vi "GrapgicalLec2.vi"() -> ()   [LabVIEW 2018]
panel:
  in  "Stop Button":bool
  out "String 3":string
  in  "a":dbl
  in  "stop 2":bool
  out "Boolean 5":bool
  out "Boolean 4":bool
  in  "LED 2":bool
  in  "LED 1":bool
  in  "stop":bool
  out "Boolean 2":bool
  in  "Boolean":bool
  out "XY Graph 2":cluster{dbl[], dbl[]}(graph)
  out "XY Graph":cluster{dbl[], dbl[]}(graph)
  out "1 root":bool
  out "2 roots":bool
  out "String":string
  in  "Numeric":dbl
  out "?":dbl
  in  "Focal Length":dbl
  in  "Polarization":dbl(knob) min=0.0 max=90.0 step=5.0 scale=0.0..90.0
  in  "Wavelength":dbl
  in  "Numeric Aperature":dbl
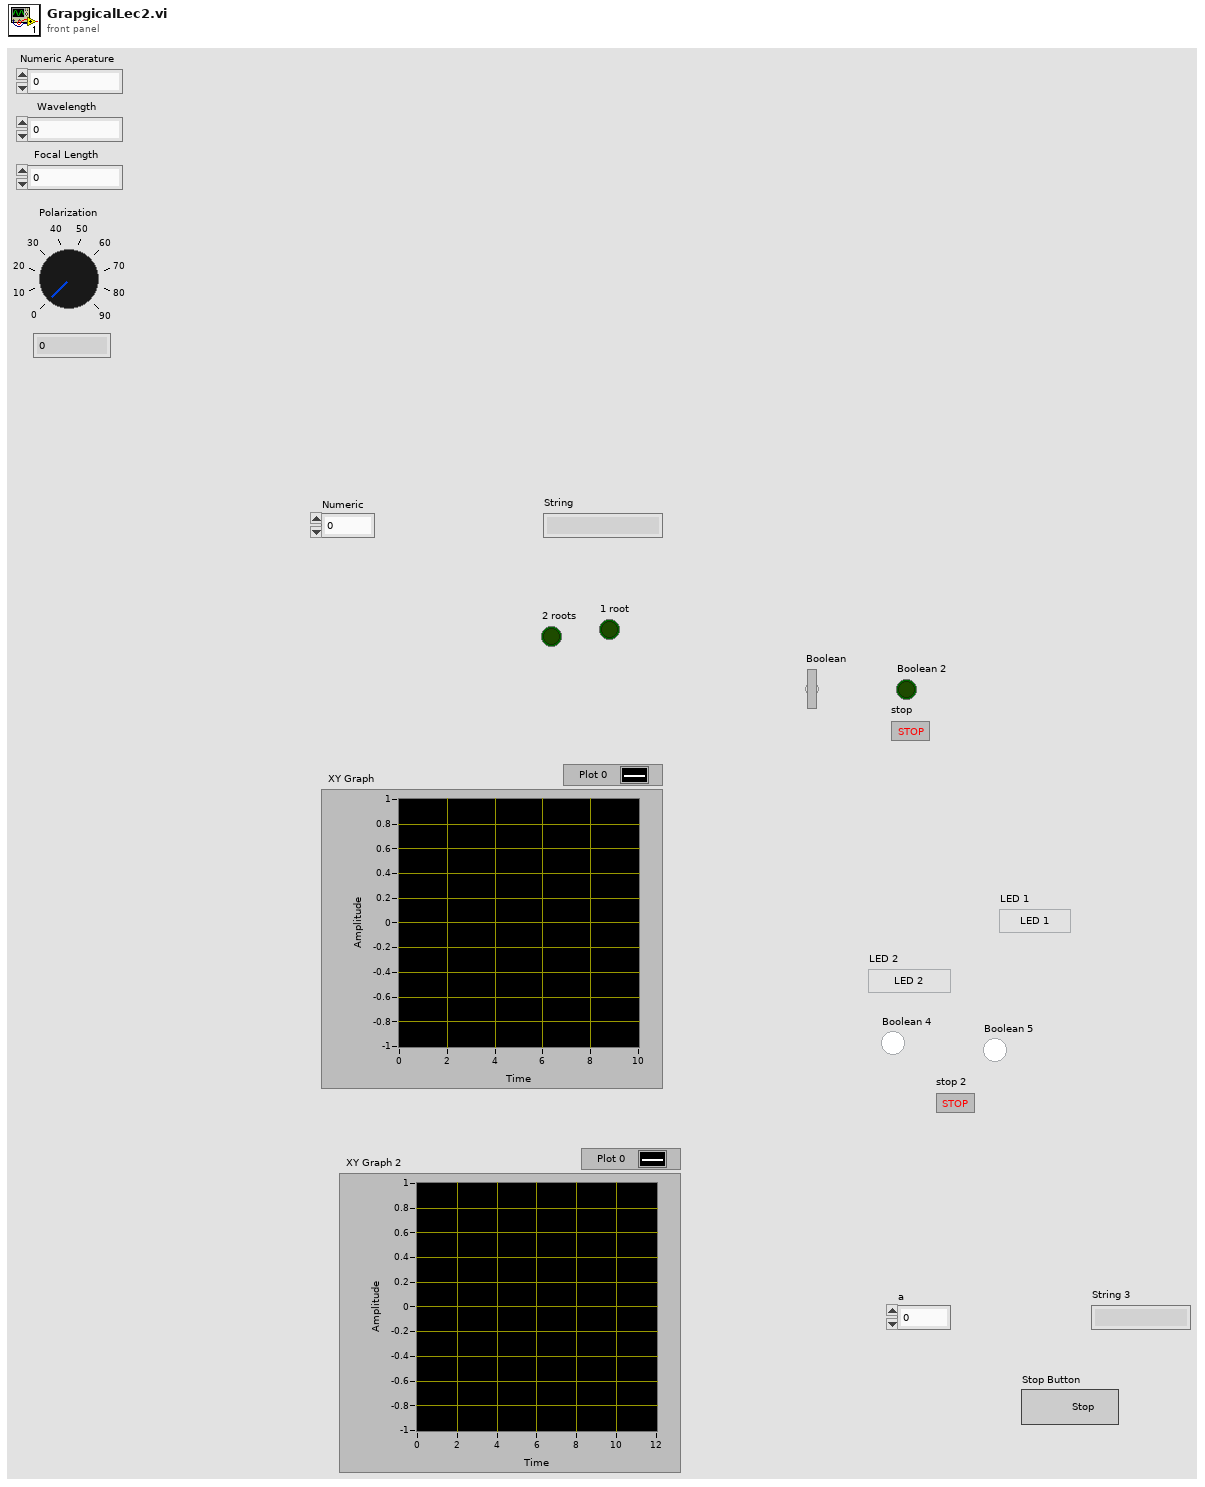
[diagram p1: front panel]
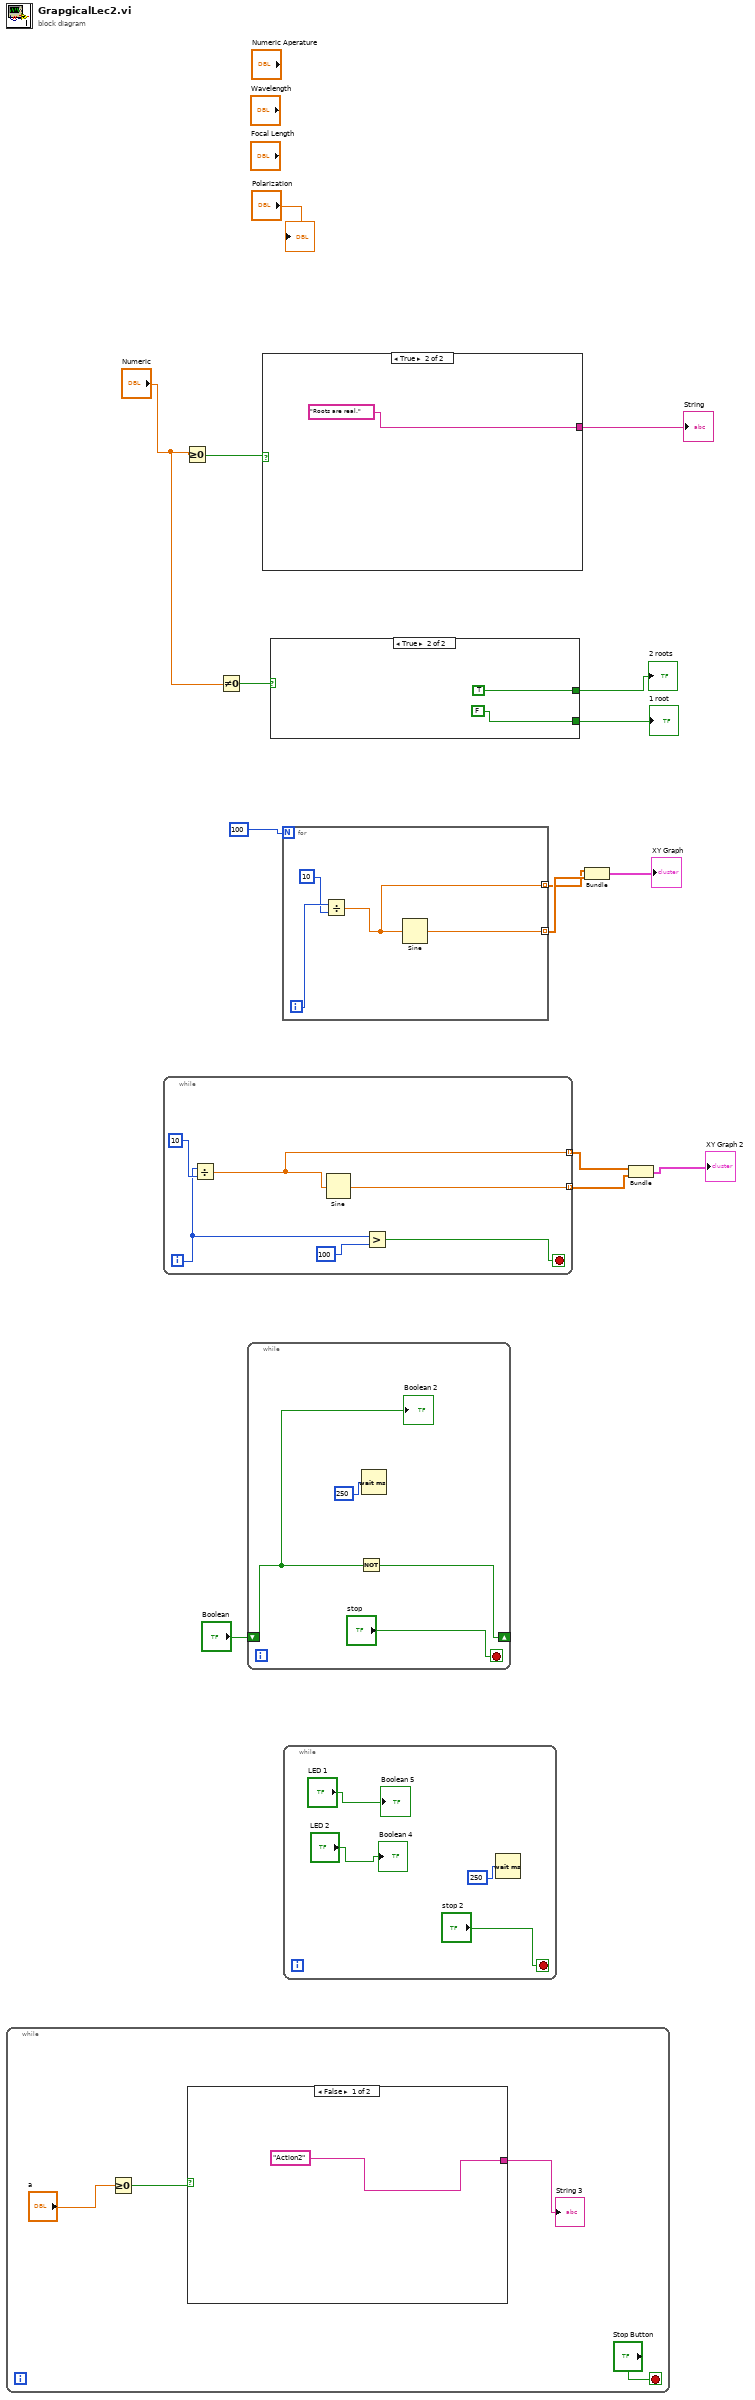
[diagram p0: block diagram]
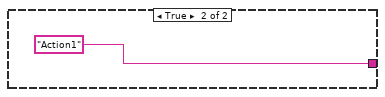
[diagram p2: hidden frame]
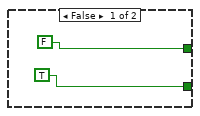
[diagram p3: hidden frame]
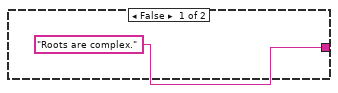
[diagram p4: hidden frame]
diagram:
  n1 = while {
    stop <- "Stop Button" stop-if-true
    n2 = Greater Or Equal To 0?(x="a") -> (x >= 0?=w17:bool)
    n3 = case shown="False" w17 {
      tunnel: ["Action2" "Action1"] -> w18
      frame False {
      }
      frame True {
      }
    }
    "String 3" <- w18
  }
  n4 = while {
    tunnel: [w23] -> w3 mode=indexing
    tunnel: [w22] -> w4 mode=indexing
    i -> [w26]
    stop <- w24 stop-if-true
    n5 = Divide(x=w26, y=10) -> (x/y=w22:dbl)
    n6 = Sine(x=w22) -> (sin(x)=w23:dbl)
    n7 = Greater?(x=w26, y=100) -> (0:w24:bool)
  }
  n8 = Greater Or Equal To 0?(x="Numeric") -> (x >= 0?=w13:bool)
  n9 = Not Equal To 0?(x="Numeric") -> (x != 0?=w11:bool)
  n10 = while {
    shift-right: [w30] -> _
    shift-left: "Boolean" -> [w29]
    stop <- "stop" stop-if-true
    n11 = Not(x=w29) -> (.not. x?=w30:bool)
    n12 = Wait (ms)(milliseconds to wait=250) -> ()  [unwired: 1 out]
    "Boolean 2" <- w29
  }
  n13 = case shown="True" w13 {
    tunnel: ["Roots are complex." "Roots are real."] -> w14
    frame False {
    }
    frame True {
    }
  }
  "String" <- w14
  n14 = case shown="True" w11 {
    tunnel: [FALSE TRUE] -> w10
    tunnel: [TRUE FALSE] -> w9
    frame False {
    }
    frame True {
    }
  }
  "2 roots" <- w10
  "1 root" <- w9
  n15 = for {
    N: 100 -> [_]
    tunnel: [w41] -> w7 mode=indexing
    tunnel: [w40] -> w6 mode=indexing
    i -> [w39]
    n16 = Divide(x=w39, y=10) -> (x/y=w40:dbl)
    n17 = Sine(x=w40) -> (sin(x)=w41:dbl)
  }
  n18 = while {
    stop <- "stop 2" stop-if-true
    n19 = Wait (ms)(milliseconds to wait=250) -> ()  [unwired: 1 out]
    "Boolean 5" <- "LED 1"
    "Boolean 4" <- "LED 2"
  }
  n20 = Bundle(w6, w7) -> (→"XY Graph":cluster{dbl[], dbl[]})  [unwired: 1 in]
  n21 = Bundle(w4, w3) -> (→"XY Graph 2":cluster{dbl[], dbl[]})  [unwired: 1 in]
  "?" <- "Polarization"
